vi "SetLastSelectedRowIndex.vi"(0 "reference in":refnum<class "DataGridView.lvclass">, 5 "LastSelectedRowIndex":i32=-1, 11 "error in (no error)":errorcluster) -> (4 "reference out":refnum<class "DataGridView.lvclass">, 15 "error out":errorcluster)   [LabVIEW 2018, in "DataGridView.lvclass"]
doc: "Sets the LastSelectedRowIndex, if nothing was selected use -1"
uses:
  DataGridView.lvclass
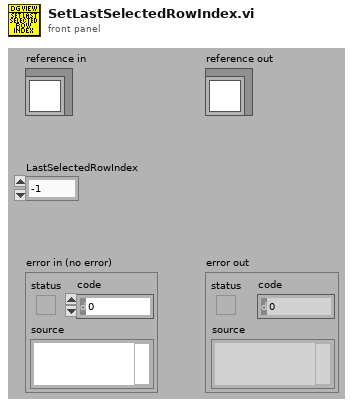
[diagram p1: front panel]
types:
  T1 = typedef "DataGridView.lvclass/ObjectAttributes.ctl" = cluster{"DataGridView":refnum<k24>, "SelectionChangedEvent":refnum<user-event>, "SelectionChanged callback ref":refnum<k27>, "LastSelectedRowIndex":i32}
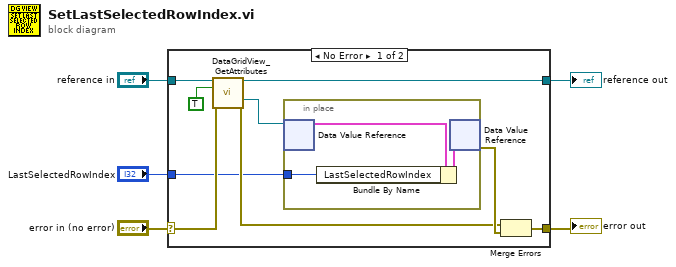
[diagram p0: block diagram]
diagram:
  n1 = case shown="No Error" "error in (no error)" {
    selector: "error in (no error)" -> [w9 w19]
    tunnel: [w13 w19] -> w4
    tunnel: [w11 w18] -> w2
    tunnel: "reference in" -> [w12 w18]
    tunnel: "LastSelectedRowIndex" -> [w6 _]
    frame No Error {
      n2 = call "DataGridView_GetAttributes.vi"("reference in"=w12, "OnlyGetDvrReference(False)"=TRUE, "error in (no error)"=w9) -> ("reference out"=w11:refnum<class "DataGridView.lvclass">, "DataRef"=w10:refnum<data-value>, "error out"=w8:errorcluster)  [unwired: 9 in, 1 out]
      n3 = in-place {
        in-place-border: w6 -> [w17]
        n4 = in-place-dvr #1(w10) -> (w16:T1)  [unwired: 1 out]
        n5 = Bundle By Name(cluster=w16, "LastSelectedRowIndex"=w17) -> (w15:T1)
        n6 = in-place-dvr #1(w15) -> (w14:errorcluster)  [unwired: 1 out]
      }
      n7 = Merge Errors(w8, w14) -> (w13:errorcluster)
    }
    frame Error {
    }
  }
  "error out" <- w4
  "reference out" <- w2
